vi "Create Do Cmd.vi"(0 "#DO":u8, 5 "value":bool, 7 "Time uSec":u32) -> (4 "Numeric":u64)   [LabVIEW 2019]
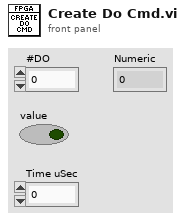
[diagram p1: front panel]
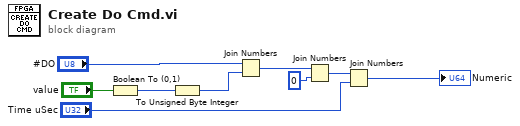
[diagram p0: block diagram]
diagram:
  n1 = Boolean To (0,1)(Boolean="value") -> (0, 1=w6:i16)
  n2 = To Unsigned Byte Integer(number=w6) -> (unsigned 8bit integer=w5:u8)
  n3 = Join Numbers(hi="#DO", lo=w5) -> ((hi.lo)=w4:u16)
  n4 = Join Numbers(hi=w4, lo=u16 0) -> ((hi.lo)=w3:u32)
  n5 = Join Numbers(hi=w3, lo="Time uSec") -> ((hi.lo)=→"Numeric":u64)
